vi "Scan Engine.vi"() -> ()   [LabVIEW 2017]
uses:
  Controls/System Parameters.ctl
  Hardware/Table Stage/Controls/Translation Stage Cluster.ctl
  Controls/Translation Stage Types.ctl
  Controls/QueueNames.ctl
  Controls/Queue Manager Actions.ctl
  Controls/MessagePacket.ctl
panel:
  in  "Slice pattern":T1={"repitition"=14, "thick slice (um)"=500.0, "thin slice (um)"=100.0} {"thin slice (um)" format="%#_13g"; "thick slice (um)" format="%#_13g"}
  out "Error Out":errorcluster
  in  "System Parameters":T2={"Vibratome"={"Z Bottom [mm]"=0.0, "Pre Cut Dwell [s]"=1.0, "Blade Frequency [RPM]"=3000, "Slice Speed [mm/s]"=0.1, "Post Cut Dwell [s]"=1.0, "Ramp Time [s]"=0.5, "Start X [mm]"=118.7, "Start Y [mm]"=81.6, "Slice Length [mm]"=25.0, "Slice Axis"=enum."X Axis", "Controller VISA Ref"="COM3"}, "Table Stages"={"X Stage"={"Position"=0.0, "Is.Enabled?"=FALSE, "Is.Connected?"=FALSE, "Device SN"="45876060", "AccelerationMaximum"=50.0, "VelocityMaximum"=50.0, "Acceleration"=10.0, "Velocity"=10.0, "waitTimeout (ms)"=1000000, "Model"=enum."Thorlabs LTS", "Is.Homed?"=FALSE}, "Y Stage"={"Position"=0.0, "Is.Enabled?"=FALSE, "Is.Connected?"=FALSE, "Device SN"="45875512", "AccelerationMaximum"=50.0, "VelocityMaximum"=50.0, "Acceleration"=10.0, "Velocity"=10.0, "waitTimeout (ms)"=1000000, "Model"=enum."Thorlabs LTS", "Is.Homed?"=FALSE}, "Z Stage"={"Position"=0.0, "Is.Enabled?"=FALSE, "Is.Connected?"=FALSE, "Device SN"="49872414", "AccelerationMaximum"=0.1, "VelocityMaximum"=0.1, "Acceleration"=0.1, "Velocity"=0.1, "waitTimeout (ms)"=100000, "Model"=enum."Thorlabs MLJ", "Is.Homed?"=FALSE}}}
  in  "Imaging Parameters":T5={"Save Path"=path "E:/Jiarui/0405volume", "# Cscan"=1, "ROI Parameters"={"ROI (mm)"={"X (mm)"=1.0, "Y (mm)"=1.0}, "Shift (mm)"={"Xshift (mm)"=0.0, "Yshift (mm)"=0.0}}, "Scan Parameters"={"# Scan"={"#Ascan"=400, "#Bscan"=400}, "# Rpt"={"#ARpt"=1, "#BRpt"=1}, "Aline Rate"=2, "# Extra"={"# ARpt_extra"=5, "#Brtn_extra"=80}}, "Objective"=1, "Image Index"=0} {"Objective" items=["5X LKM05", "10X LKM10", "20X LKM20", "10X LSM02"]; "Scan Parameters"."Aline Rate" items=["76 KHz", "146 KHz", "76 KHz", "28 KHz", "10 KHz"]}
  in  "Mosaic Parameters":T6={"Overlap Options"={"Overlap Type"=enum."No Overlap", "Percent Overlap"=0, "Justify"=enum."Start"}, "Mosaic Range"={"X Axis"={"Start [mm]"=49.3, "Steps [pts]"=25, "End [mm]"=61.3}, "Y Axis"={"Start [mm]"=69.6, "Steps [pts]"=26, "End [mm]"=82.1}}, "Scan Pattern"=enum."Uni-directional", "Number of slices"=30}
  in  "Error In":errorcluster
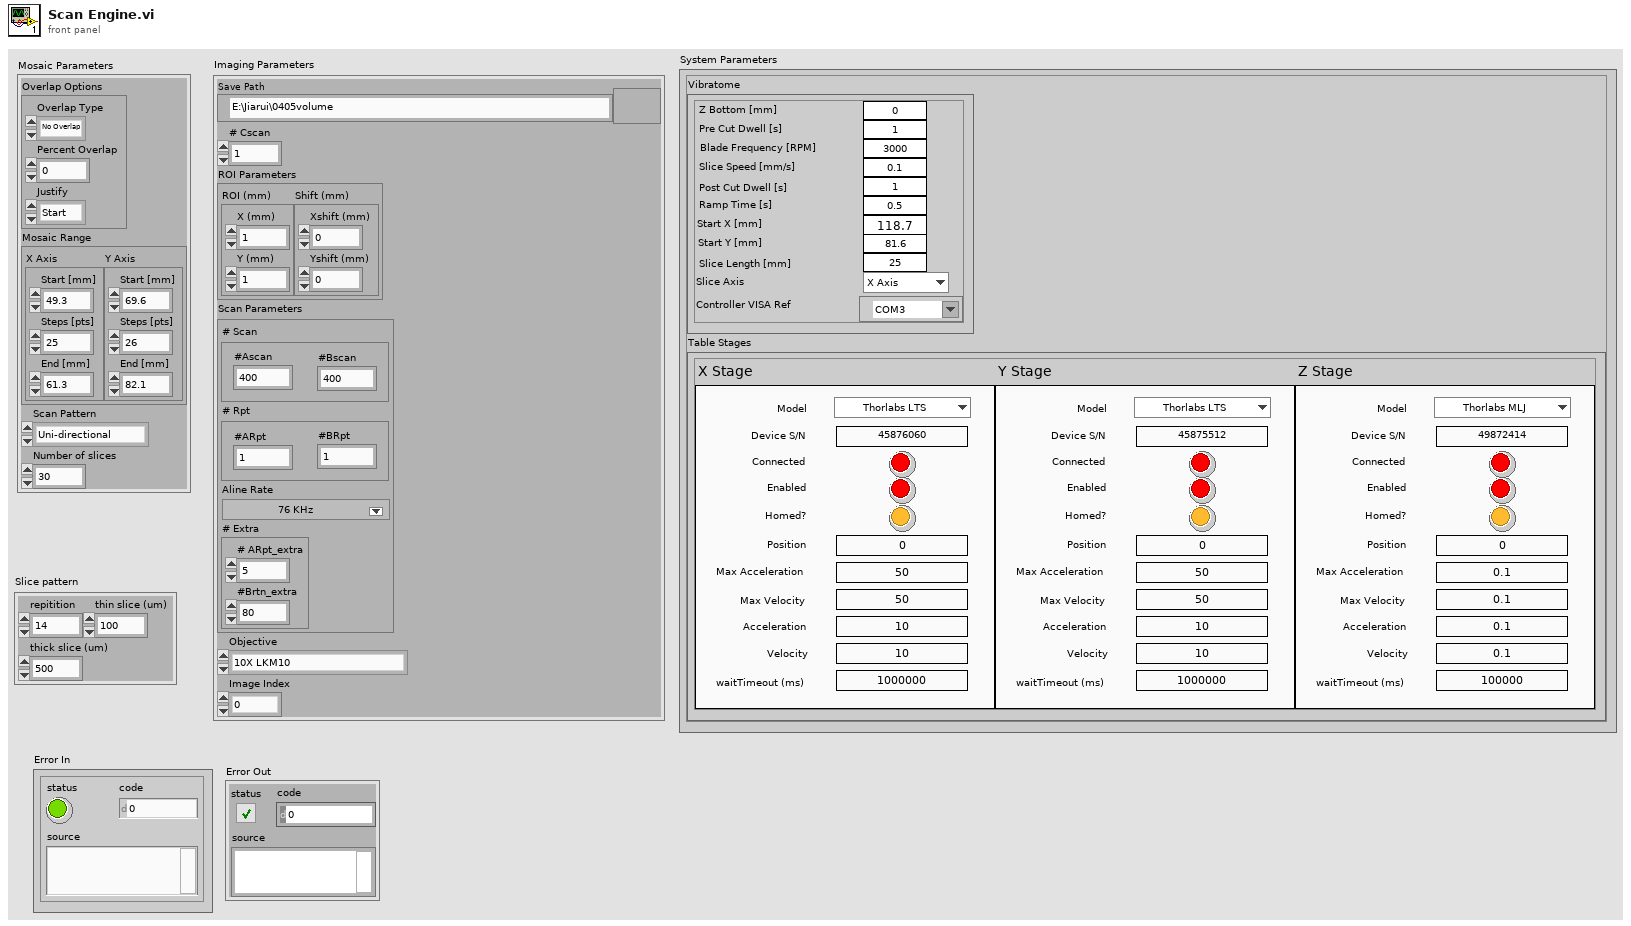
[diagram p1: front panel]
types:
  T1 = cluster{"repitition":i32, "thick slice (um)":dbl, "thin slice (um)":dbl}
  T2 = typedef "System Parameters.ctl" = cluster{"Vibratome":cluster{"Z Bottom [mm]":dbl, "Pre Cut Dwell [s]":dbl, "Blade Frequency [RPM]":u16, "Slice Speed [mm/s]":dbl, "Post Cut Dwell [s]":dbl, "Ramp Time [s]":dbl, "Start X [mm]":dbl, "Start Y [mm]":dbl, "Slice Length [mm]":dbl, "Slice Axis":enum16{"X Axis", "Y Axis", "Z Axis"}, "Controller VISA Ref":refnum<visa-resource-name>}, "Table Stages":cluster{"X Stage":T3, "Y Stage":T3, "Z Stage":T3}}
  T3 = typedef "Translation Stage Cluster.ctl" = cluster{"Position":dbl, "Is.Enabled?":bool, "Is.Connected?":bool, "Device SN":string, "AccelerationMaximum":dbl, "VelocityMaximum":dbl, "Acceleration":dbl, "Velocity":dbl, "waitTimeout (ms)":i32, "Model":T4, "Is.Homed?":bool}
  T4 = typedef "Translation Stage Types.ctl" = enum16{"None", "Thorlabs LTS", "Thorlabs MLJ"}
  T5 = cluster{"Save Path":path, "# Cscan":i32, "ROI Parameters":cluster{"ROI (mm)":cluster{"X (mm)":sgl, "Y (mm)":sgl}, "Shift (mm)":cluster{"Xshift (mm)":sgl, "Yshift (mm)":sgl}}, "Scan Parameters":cluster{"# Scan":cluster{"#Ascan":i32, "#Bscan":i32}, "# Rpt":cluster{"#ARpt":i32, "#BRpt":i32}, "Aline Rate":u16, "# Extra":cluster{"# ARpt_extra":i32, "#Brtn_extra":i32}}, "Objective":u16, "Image Index":i16}
  T6 = cluster{"Overlap Options":cluster{"Overlap Type":enum16{"No Overlap", "X Only", "Y Only", "X and Y"}, "Percent Overlap":u8, "Justify":enum16{"Start", "Center", "End"}}, "Mosaic Range":cluster{"X Axis":cluster{"Start [mm]":dbl, "Steps [pts]":u16, "End [mm]":dbl}, "Y Axis":cluster{"Start [mm]":dbl, "Steps [pts]":u16, "End [mm]":dbl}}, "Scan Pattern":enum16{"Uni-directional", "Bi-Directional", "Spiral Out", "Spiral In"}, "Number of slices":i16}
  T7 = typedef "MessagePacket.ctl" = cluster{"Message":string, "Parameter":variant}
  T8 = typedef "Queue Manager Actions.ctl" = enum16{"Init", "Enqueue", "Enqueue All", "Preview Queue", "Dequeue", "Get Status", "Flush Queue", "Flush All Queues", "Release All Queues", "Release Queue", "Enqueue at Opposite End"}
  T9 = typedef "QueueNames.ctl" = enum16{"Main GUI", "Main Scan Processor", "Main Display", "Main Table Stage GUI", "Main Table Stage Proc.", "Scan Engine", "Vibratome GUI", "Vibratome Processor", "Slice Engine"}
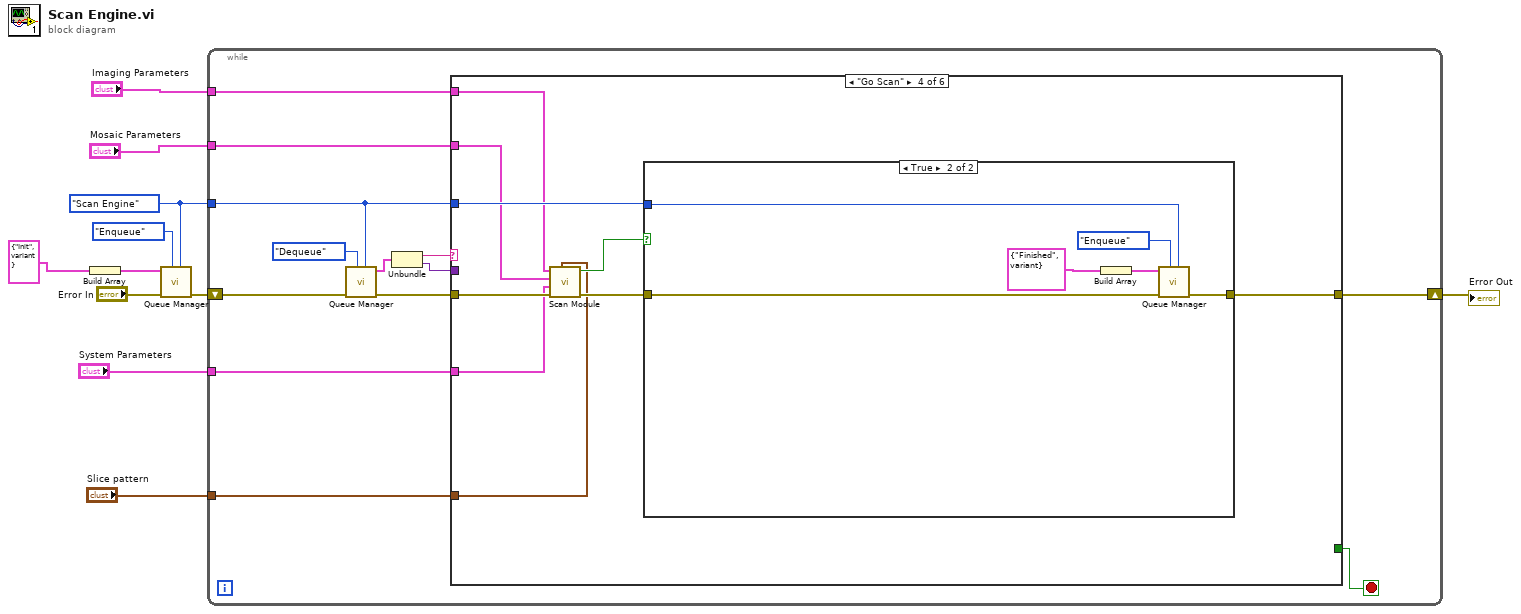
[diagram p0: block diagram]
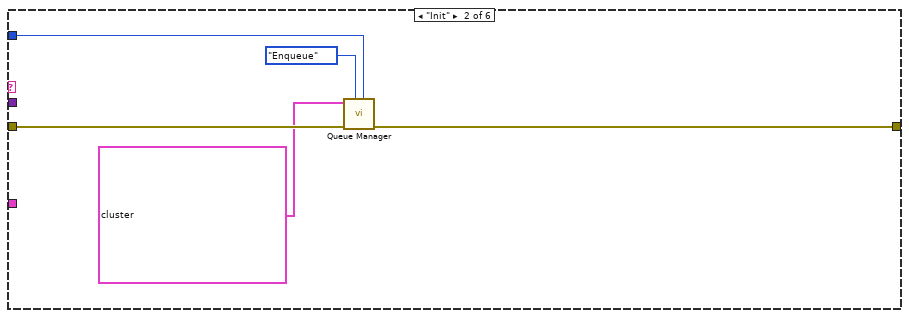
[diagram p3: hidden frame]
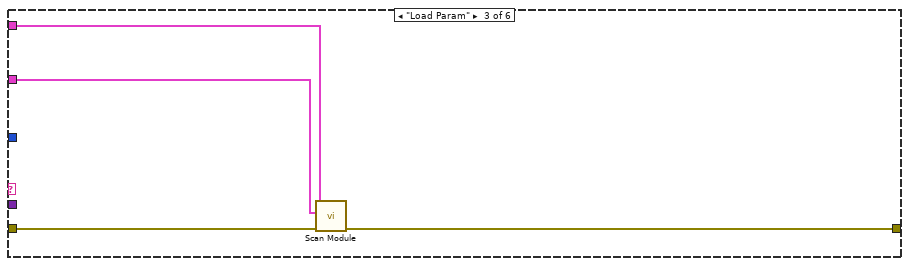
[diagram p4: hidden frame]
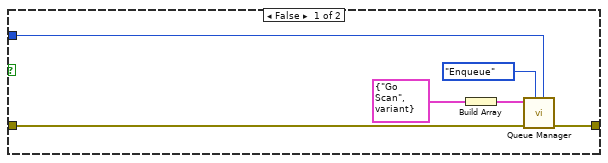
[diagram p5: hidden frame]
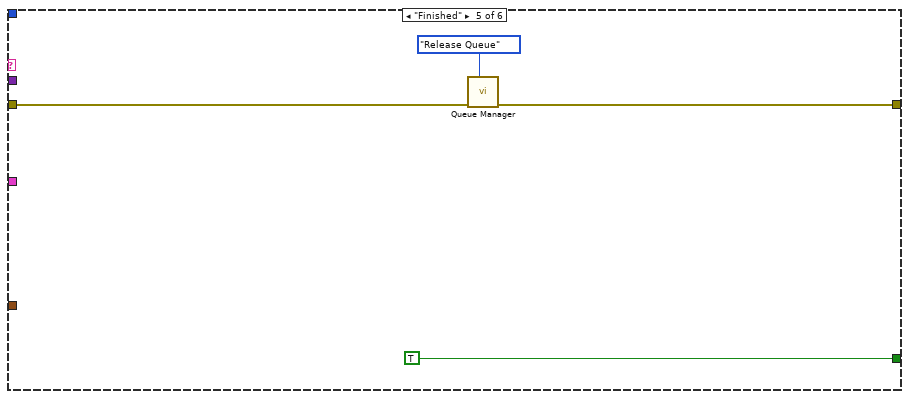
[diagram p6: hidden frame]
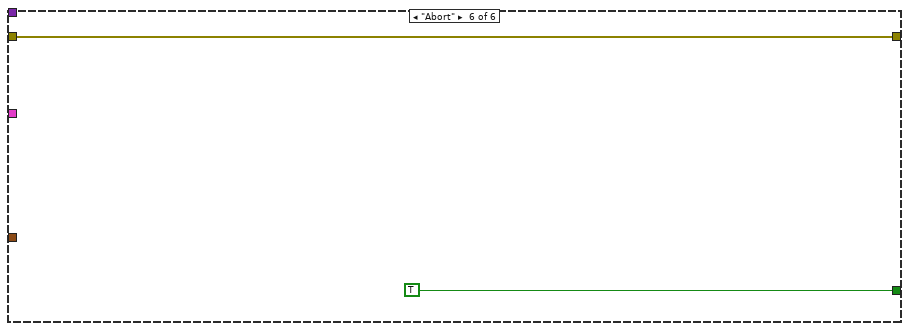
[diagram p7: hidden frame]
diagram:
  w6 = QueueNames."Scan Engine" ("Queue Name")
  n1 = Build Array(T7 {"Message"="Init", "Parameter"=variant} ("Message Packet")) -> (w7:T7[])
  n2 = call "Queue Manager.vi"("Queue Name"=w6, "Action"=Queue_Manager_Actions."Enqueue", "Error In"="Error In", "Message Packet Array"=w7) -> ("Error Out"=w9:errorcluster)  [unwired: 3 in, 4 out]
  n3 = while {
    tunnel: w6 -> [w16]
    shift-right: [w17] -> w3
    shift-left: w9 -> [w24]
    tunnel: "Mosaic Parameters" -> [w15]
    tunnel: "Imaging Parameters" -> [w14]
    tunnel: "System Parameters" -> [w13]
    tunnel: "Slice pattern" -> [w12]
    stop <- w21 stop-if-true
    n4 = call "Queue Manager.vi"("Queue Name"=w16, "Action"=Queue_Manager_Actions."Dequeue", "Error In"=w24) -> ("Error Out"=w18:errorcluster, "Message Packet [Out]"=w22:T7)  [unwired: 4 in, 3 out]
    n5 = Unbundle(w22) -> ("Message"=w20:string, "Parameter"=w19:variant)
    n6 = case shown="\"Go Scan\"" w20 {
      tunnel: [_ _ _ _ TRUE TRUE] -> w21
      tunnel: w19 -> [_ _ _ _ _ _]
      tunnel: w18 -> [w25 w30 w34 w43 w57 w60]
      tunnel: [w25 w29 w33 w41 w56 w60] -> w17
      tunnel: w16 -> [_ w28 _ w40 _ _]
      tunnel: w15 -> [_ _ w32 w37 _ _]
      tunnel: w14 -> [_ _ w31 w38 _ _]
      tunnel: w13 -> [_ _ _ w36 _ _]
      tunnel: w12 -> [_ _ _ w35 _ _]
      frame "Error", Default {
      }
      frame "Init" {
        n7 = call "Queue Manager.vi"("Queue Name"=w28, "Action"=Queue_Manager_Actions."Enqueue", "Error In"=w30, "Message Packet Array"=T7[] [{"Message"="Load Param", "Parameter"=variant}, {"Message"="Go Scan", "Parameter"=variant}]) -> ("Error Out"=w29:errorcluster)  [unwired: 3 in, 4 out]
      }
      frame "Load Param" {
        n8 = call "Scan Module.vi"("Error In"=w34, "Mosaic Parameters"=w32, "Imaging Parameters"=w31) -> ("Error Out"=w33:errorcluster)  [unwired: 7 in, 1 out]
      }
      frame "Go Scan" {
        n9 = call "Scan Module.vi"("Slice pattern"=w35, "Error In"=w43, "System Parameters"=w36, "Mosaic Parameters"=w37, "Imaging Parameters"=w38) -> ("Error Out"=w39:errorcluster, "Finished?"=w42:bool)  [unwired: 5 in]
        n10 = case shown="True" w42 {
          tunnel: w39 -> [w49 w55]
          tunnel: [w48 w54] -> w41
          tunnel: w40 -> [w47 w53]
          frame False {
            n11 = Build Array(T7 {"Message"="Go Scan", "Parameter"=variant} ("Message Packet")) -> (w44:T7[])
            n12 = call "Queue Manager.vi"("Queue Name"=w47, "Action"=Queue_Manager_Actions."Enqueue", "Error In"=w49, "Message Packet Array"=w44) -> ("Error Out"=w48:errorcluster)  [unwired: 3 in, 4 out]
          }
          frame True {
            n13 = Build Array(T7 {"Message"="Finished", "Parameter"=variant} ("Message Packet")) -> (w50:T7[])
            n14 = call "Queue Manager.vi"("Queue Name"=w53, "Action"=Queue_Manager_Actions."Enqueue", "Error In"=w55, "Message Packet Array"=w50) -> ("Error Out"=w54:errorcluster)  [unwired: 3 in, 4 out]
          }
        }
      }
      frame "Finished" {
        n15 = call "Queue Manager.vi"("Action"=Queue_Manager_Actions."Release Queue", "Error In"=w57) -> ("Error Out"=w56:errorcluster)  [unwired: 5 in, 4 out]
      }
      frame "Abort" {
      }
    }
  }
  "Error Out" <- w3
